vi "lib_mpfit_parse_return.vi"(11 "return code":i32) -> (1 "success":bool, 2 "exit message":string)   [LabVIEW 2017]
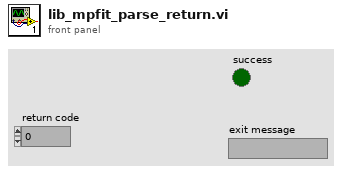
[diagram p1: front panel]
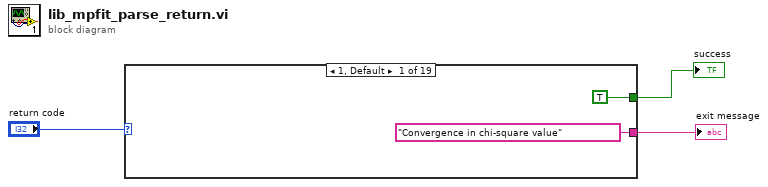
[diagram p0: block diagram]
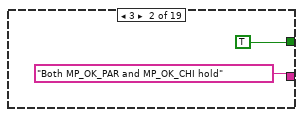
[diagram p2: hidden frame]
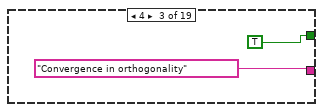
[diagram p3: hidden frame]
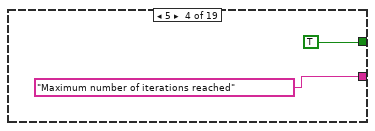
[diagram p4: hidden frame]
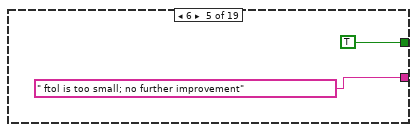
[diagram p5: hidden frame]
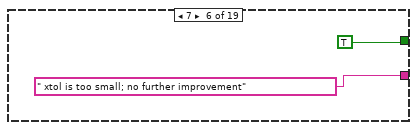
[diagram p6: hidden frame]
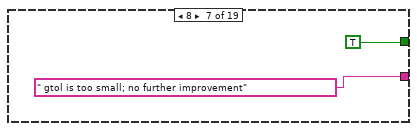
[diagram p7: hidden frame]
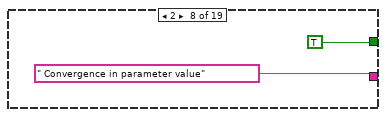
[diagram p8: hidden frame]
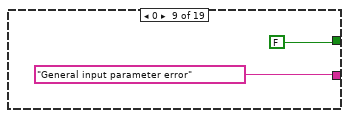
[diagram p9: hidden frame]
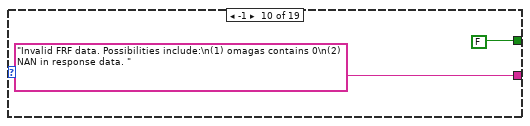
[diagram p10: hidden frame]
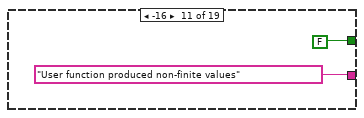
[diagram p11: hidden frame]
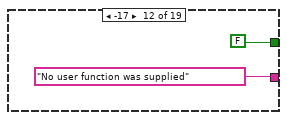
[diagram p12: hidden frame]
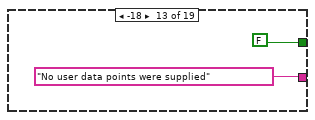
[diagram p13: hidden frame]
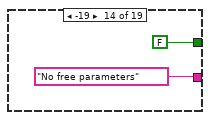
[diagram p14: hidden frame]
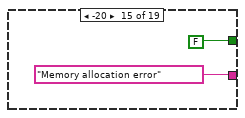
[diagram p15: hidden frame]
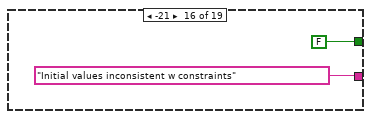
[diagram p16: hidden frame]
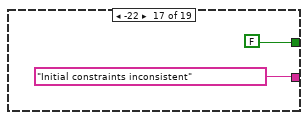
[diagram p17: hidden frame]
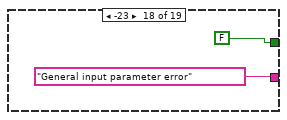
[diagram p18: hidden frame]
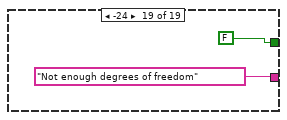
[diagram p19: hidden frame]
diagram:
  n1 = case shown="1, Default" "return code" {
    tunnel: ["Convergence in chi-square value" ("error message (\"\")") "Both MP_OK_PAR and MP_OK_CHI hold" ("error message (\"\")") "Convergence in orthogonality" ("error message (\"\")") "Maximum number of iterations reached" ("error message (\"\")") " ftol is too small; no further improvement" ("error message (\"\")") " xtol is too small; no further improvement" ("error message (\"\")") " gtol is too small; no further improvement" ("error message (\"\")") " Convergence in parameter value" ("error message (\"\")") "General input parameter error" ("error message (\"\")") "Invalid FRF data. Possibilities include:\n(1) omagas contains 0\n(2) NAN in response data. " ("error message (\"\")") "User function produced non-finite values" ("error message (\"\")") "No user function was supplied" ("error message (\"\")") "No user data points were supplied" ("error message (\"\")") "No free parameters" ("error message (\"\")") "Memory allocation error" ("error message (\"\")") "Initial values inconsistent w constraints" ("error message (\"\")") "Initial constraints inconsistent" ("error message (\"\")") "General input parameter error" ("error message (\"\")") "Not enough degrees of freedom" ("error message (\"\")")] -> w2
    tunnel: [TRUE TRUE TRUE TRUE TRUE TRUE TRUE TRUE FALSE FALSE FALSE FALSE FALSE FALSE FALSE FALSE FALSE FALSE FALSE] -> w1
    frame 1, Default {
    }
    frame 3 {
    }
    frame 4 {
    }
    frame 5 {
    }
    frame 6 {
    }
    frame 7 {
    }
    frame 8 {
    }
    frame 2 {
    }
    frame 0 {
    }
    frame -1 {
    }
    frame -16 {
    }
    frame -17 {
    }
    frame -18 {
    }
    frame -19 {
    }
    frame -20 {
    }
    frame -21 {
    }
    frame -22 {
    }
    frame -23 {
    }
    frame -24 {
    }
  }
  "exit message" <- w2
  "success" <- w1
